vi "Version_4.9_8_on-chip_valves_for25ulSyringe_withModfied_Plunging.vi"() -> ()   [LabVIEW 2020] (continued)
                    n8528 = Wait (ms)(milliseconds to wait=w300) -> ()  [unwired: 1 out]
                  }
                  frame #3 {
                    n8529 = local write "Suction On/Off"(TRUE ("Suction On/Off")) -> ()
                  }
                  frame #4 {
                    n8530 = local read "Delay before\n1st movement\nof grid"() -> (w304:dbl)
                    n8531 = Wait (ms)(milliseconds to wait=w304) -> ()  [unwired: 1 out]
                  }
                  frame #5 {
                    n8532 = local read "No of cycles\nof up-down\nmovement"() -> (w305:dbl)
                    n8533 = for {
                      N: w305 -> [_]
                      shift-right: [w319] -> w311
                      shift-left: w313 -> [w321]
                      shift-right: [w318] -> w310
                      shift-left: w312 -> [w320]
                      shift-right: [w315] -> w307
                      shift-left: w309 -> [w317]
                      shift-right: [w314] -> w306
                      shift-left: w308 -> [w316]
                      n8534 = stacked-sequence {
                        seq-local: [w323 _ _ _ _ _] -> [_ _ _ w345 _ _]
                        seq-local: [w322 _ _ _ _ _] -> [_ _ _ w344 _ _]
                        seq-local: [_ _ w329 _ _ _] -> [_ _ _ _ _ w353]
                        seq-local: [_ _ w328 _ _ _] -> [_ _ _ _ _ w352]
                        tunnel: [_ _ _ w346 _ _] -> w319
                        tunnel: [_ _ _ w348 _ _] -> w318
                        tunnel: w321 -> [w326 _ _ _ _ _]
                        tunnel: w320 -> [w325 _ _ _ _ _]
                        tunnel: w317 -> [_ _ w331 _ _ _]
                        tunnel: w316 -> [_ _ w330 _ _ _]
                        tunnel: [_ _ _ _ _ w351] -> w315
                        tunnel: [_ _ _ _ _ w350] -> w314
                        frame #0 {
                          n8535 = VISA Write(VISA resource name=w326, write buffer="d", error in (no error)=w325) -> (VISA resource name out=w323:refnum<visa-resource-name>, error out=w322:errorcluster)  [unwired: 1 out]
                        }
                        frame #1 {
                          n8536 = local read "Duration for \nup/down\nMovement of Grid"() -> (w327:u32)
                          n8537 = Wait (ms)(milliseconds to wait=w327) -> ()  [unwired: 1 out]
                        }
                        frame #2 {
                          n8538 = stacked-sequence {
                            tunnel: w331 -> [_ w339 _]
                            tunnel: w330 -> [_ w338 _]
                            tunnel: [_ w337 _] -> w329
                            tunnel: [_ w336 _] -> w328
                            frame #0 {
                              n8539 = local read "Translation Step SIze\nwhile plunging"() -> (w332:dbl)
                              n8540 = local read "k1"() -> (w334:dbl)
                              n8541 = Decrement(x=w334) -> (x-1=w333:dbl)
                              n8542 = Multiply(x=w332, y=w333) -> (x*y=w335:dbl)
                              n8543 = local write "k2"(w333) -> ()
                              n8544 = local write "Position"(w335) -> ()
                            }
                            frame #1 {
                              w342 = 1 items=["Channel1"=1, "Channel2"=2, "Channel3"=3, "Channel4"=4] ("channel")
                              n8545 = local read "Position"() -> (w341:i32)
                              n8546 = invoke class="KCubeInertialMotor" method="MoveTo"(reference=w339, error in=w338, "channel"=w342, "position"=w341, "waitTimeout"=10000) -> (reference out=w337:refnum<k24>, error out=w336:errorcluster)  [unwired: 1 in, 4 out]
                            }
                            frame #2 {
                              n8547 = local read "Wait time for\ntranslation"() -> (w343:u32)
                              n8548 = Wait (ms)(milliseconds to wait=w343) -> ()  [unwired: 1 out]
                            }
                          }
                        }
                        frame #3 {
                          n8549 = VISA Write(VISA resource name=w345, write buffer="u", error in (no error)=w344) -> (VISA resource name out=w346:refnum<visa-resource-name>, error out=w348:errorcluster)  [unwired: 1 out]
                        }
                        frame #4 {
                          n8550 = local read "Duration for \nup/down\nMovement of Grid"() -> (w349:u32)
                          n8551 = Wait (ms)(milliseconds to wait=w349) -> ()  [unwired: 1 out]
                        }
                        frame #5 {
                          n8552 = stacked-sequence {
                            tunnel: w353 -> [_ w361 _]
                            tunnel: w352 -> [_ w360 _]
                            tunnel: [_ w359 _] -> w351
                            tunnel: [_ w358 _] -> w350
                            frame #0 {
                              n8553 = local read "Translation Step SIze\nwhile plunging"() -> (w354:dbl)
                              n8554 = local read "k2"() -> (w356:dbl)
                              n8555 = Increment(x=w356) -> (x+1=w355:dbl)
                              n8556 = Multiply(x=w354, y=w355) -> (x*y=w357:dbl)
                              n8557 = local write "k1"(w355) -> ()
                              n8558 = local write "Position"(w357) -> ()
                            }
                            frame #1 {
                              w364 = 1 items=["Channel1"=1, "Channel2"=2, "Channel3"=3, "Channel4"=4] ("channel")
                              n8559 = local read "Position"() -> (w363:i32)
                              n8560 = invoke class="KCubeInertialMotor" method="MoveTo"(reference=w361, error in=w360, "channel"=w364, "position"=w363, "waitTimeout"=10000) -> (reference out=w359:refnum<k24>, error out=w358:errorcluster)  [unwired: 1 in, 4 out]
                            }
                            frame #2 {
                              n8561 = local read "Wait time for\ntranslation"() -> (w365:u32)
                              n8562 = Wait (ms)(milliseconds to wait=w365) -> ()  [unwired: 1 out]
                            }
                          }
                        }
                      }
                    }
                  }
                  frame #6 {
                    n8563 = VISA Write(VISA resource name=w370, write buffer="p", error in (no error)=w369) -> (VISA resource name out=w368:refnum<visa-resource-name>, error out=w367:errorcluster)  [unwired: 1 out]
                    n8564 = local write "Suction On/Off"(FALSE ("Suction On/Off")) -> ()
                  }
                }
              }
              frame "Spread the deposited protein on the grid in One Line and plunge" {
                n8565 = stacked-sequence {
                  seq-local: [_ _ _ w385 _] -> [_ _ _ _ w402]
                  seq-local: [_ _ _ w384 _] -> [_ _ _ _ w401]
                  tunnel: [_ _ _ _ w400] -> w377
                  tunnel: [_ _ _ _ w399] -> w376
                  tunnel: w375 -> [_ _ _ w387 _]
                  tunnel: w374 -> [_ _ _ w386 _]
                  frame #0 {
                    n8566 = local write "Re-deposit Sample\nonto Grid"(FALSE ("Re-deposit Sample\nonto Grid")) -> ()
                    n8567 = local write "Divert Sample \nonto Grid"(TRUE ("Divert Sample \nonto Grid")) -> ()
                    n8568 = local read "Grid Deposition\nDuration"() -> (w378:u32)
                    n8569 = Wait (ms)(milliseconds to wait=w378) -> ()  [unwired: 1 out]
                  }
                  frame #1 {
                    n8570 = local write "Suction On/Off"(TRUE ("Suction On/Off")) -> ()
                  }
                  frame #2 {
                    n8571 = local read "Delay before\n1st movement\nof grid"() -> (w382:dbl)
                    n8572 = Wait (ms)(milliseconds to wait=w382) -> ()  [unwired: 1 out]
                  }
                  frame #3 {
                    n8573 = local read "No of cycles\nof up-down\nmovement"() -> (w383:dbl)
                    n8574 = for {
                      N: w383 -> [_]
                      shift-right: [w389] -> w385
                      shift-left: w387 -> [w391]
                      shift-right: [w388] -> w384
                      shift-left: w386 -> [w390]
                      n8575 = stacked-sequence {
                        tunnel: w391 -> [w396 _]
                        tunnel: w390 -> [w395 _]
                        tunnel: [w393 _] -> w389
                        tunnel: [w392 _] -> w388
                        frame #0 {
                          n8576 = VISA Write(VISA resource name=w396, write buffer="y", error in (no error)=w395) -> (VISA resource name out=w393:refnum<visa-resource-name>, error out=w392:errorcluster)  [unwired: 1 out]
                        }
                        frame #1 {
                          n8577 = local read "Duration for \nup/down\nMovement of Grid"() -> (w397:u32)
                          n8578 = Wait (ms)(milliseconds to wait=w397) -> ()  [unwired: 1 out]
                        }
                      }
                    }
                  }
                  frame #4 {
                    n8579 = VISA Write(VISA resource name=w402, write buffer="p", error in (no error)=w401) -> (VISA resource name out=w400:refnum<visa-resource-name>, error out=w399:errorcluster)  [unwired: 1 out]
                    n8580 = local write "Suction On/Off"(FALSE ("Suction On/Off")) -> ()
                  }
                }
              }
            }
          }
          event "Set - Blotting Time": Value Change {
            n8581 = event-data() -> ()  [unwired: 1 in, 6 out]
            n8582 = local read "Blotting Time"() -> (w411:dbl)
            n8583 = Format Into String(format string="%0d", w411) -> (resulting string=w410:string)  [unwired: 2 in, 1 out]
            n8584 = Concatenate Strings("t" ("string"), w410, "\r\n") -> (w408:string)
            n8585 = VISA Write(VISA resource name=w407, write buffer=w408, error in (no error)=w406) -> (VISA resource name out=w405:refnum<visa-resource-name>, error out=w404:errorcluster)  [unwired: 1 out]
          }
          event "Set - Blotting Angle": Value Change {
            n8586 = event-data() -> ()  [unwired: 1 in, 6 out]
            n8587 = local read "Blotting Angle"() -> (w421:dbl)
            n8588 = Format Into String(format string="%0d", w421) -> (resulting string=w420:string)  [unwired: 2 in, 1 out]
            n8589 = Concatenate Strings("b" ("string"), w420, "\r\n") -> (w418:string)
            n8590 = VISA Write(VISA resource name=w417, write buffer=w418, error in (no error)=w416) -> (VISA resource name out=w415:refnum<visa-resource-name>, error out=w414:errorcluster)  [unwired: 1 out]
          }
          event "Automated Blotting \nand Plunging": Value Change {
            n8591 = event-data() -> ()  [unwired: 1 in, 6 out]
            n8592 = VISA Write(VISA resource name=w428, write buffer="z", error in (no error)=w427) -> (VISA resource name out=w425:refnum<visa-resource-name>, error out=w424:errorcluster)  [unwired: 1 out]
          }
          event "Move\nGrid Up": Value Change {
            n8593 = event-data() -> ()  [unwired: 1 in, 6 out]
            n8594 = VISA Write(VISA resource name=w431, write buffer="h", error in (no error)=w432) -> (VISA resource name out=w429:refnum<visa-resource-name>, error out=w430:errorcluster)  [unwired: 1 out]
          }
          event "Move Grid \nUp Faster": Value Change {
            n8595 = event-data() -> ()  [unwired: 1 in, 6 out]
            n8596 = VISA Write(VISA resource name=w436, write buffer="x", error in (no error)=w437) -> (VISA resource name out=w434:refnum<visa-resource-name>, error out=w435:errorcluster)  [unwired: 1 out]
          }
          event "Move\nGrid Down": Value Change {
            n8597 = event-data() -> ()  [unwired: 1 in, 6 out]
            n8598 = VISA Write(VISA resource name=w441, write buffer="l", error in (no error)=w442) -> (VISA resource name out=w439:refnum<visa-resource-name>, error out=w440:errorcluster)  [unwired: 1 out]
          }
          event "Move Grid \nDown Faster": Value Change {
            n8599 = event-data() -> ()  [unwired: 1 in, 6 out]
            n8600 = VISA Write(VISA resource name=w446, write buffer="y", error in (no error)=w447) -> (VISA resource name out=w444:refnum<visa-resource-name>, error out=w445:errorcluster)  [unwired: 1 out]
          }
          event "Stop for End of \nExperiment \nand Data Writing": Value Change {
            n8601 = event-data() -> ()  [unwired: 1 in, 6 out]
            n8602 = local read "Stop for End of \nExperiment \nand Data Writing"() -> (w453:bool)
          }
          event Timeout {
            n8603 = event-data() -> ()  [unwired: 1 in, 3 out]
          }
        }
        n8604 = property class="Instr"(reference=w124, error in=w123) -> (reference out=w125:refnum<visa-resource-name>, error out=w126:errorcluster, "Serial Settings:Number of Bytes at Serial Port"=w128:u32)
        n8605 = Greater Than 0?(x=w128) -> (x > 0?=w127:bool)
        n8606 = case shown="True" w127 {
          tunnel: [w136 w151] -> w120
          tunnel: [w135 w150] -> w122
          tunnel: w125 -> [w136 w148]
          tunnel: w126 -> [w135 w147]
          tunnel: [w134 w146] -> w121
          tunnel: w131 -> [w134 w145]
          frame False {
          }
          frame True {
            (unwired) u32 20 ("byte count")
            n8607 = VISA Read(VISA resource name=w148, byte count=16, error in (no error)=w147) -> (VISA resource name out=w151:refnum<visa-resource-name>, read buffer=w144:string, error out=w150:errorcluster)  [unwired: 1 out]
            n8608 = Spreadsheet String To Array(delimiter (Tab)=",", format string="%f", spreadsheet string=w144, array type (2D Dbl)=dbl[] []) -> (array=w140:dbl[])
            n8609 = Index Array(array=w140) -> (element #1=w137:dbl, element #2=→"Ethane Temperature":dbl)  [unwired: 2 in]
            "RH (%)" <- w137
            n8610 = call "Convert from Dynamic Data5"("Dynamic Data Type"=w137) -> ("Array"=w139:dbl[])  [unwired: 3 in]
            n8611 = call-poly <vilib>:"Append Waveforms.vi"("waveform B"=w139, "waveform A"=w145) -> ("waveform out"=w146:waveform(dbl))  [unwired: 8 in, 1 out]
            "Temperature of Ethane Graph" <- w146
          }
        }
      }
      n8612 = Merge Signals(w88, w87) -> (w89:dynamicdata)
      n8613 = call "Write To Measurement File"("Signals"=w89) -> ()  [unwired: 16 in, 3 out]
      n8614 = VISA Close(VISA resource name=w71, error in (no error)=w70) -> ()  [unwired: 1 out]
      n8615 = invoke class="KCubeInertialMotor" method="StopPolling"(reference=w84, error in=w83) -> (error out=w82:errorcluster)  [unwired: 1 in, 2 out]
      n8616 = invoke class="KCubeInertialMotorControl" method="CloseDevice"(reference=w86, error in=w82) -> ()  [unwired: 1 in, 3 out]
      "Discard fluid \nprior to 1st \ndeposition" <- FALSE ("Discard fluid \nprior to 1st \ndeposition")
      "SEC On" <- FALSE ("SEC On")
      "Affinity On" <- FALSE ("Affinity On")
      "Affinity Elution On" <- FALSE ("Affinity On")
      "Suction pressure \nfor grid deposition" <- sgl 0.0 ("Suction pressure \nfor grid deposition")
      "Net Elution \nVolume" <- 0.0 ("Net Elution \nVolume")
      "Pause Elution" <- FALSE ("Pause Elution")
    }
    frame #1 {
      # "Switch off the LEDs"
      n8617 = local write "Start the Process"(FALSE ("Start the Process")) -> ()
      n8618 = local write "Stop for End of \nExperiment \nand Data Writing"(FALSE ("Stop for End of \nExperiment \nand Data Writing")) -> ()
      n8619 = local write "Stopper that ends \nthe main loops"(FALSE ("Stopper that ends \nthe main loops")) -> ()
    }
  }
  "Volume being Injected \nin this process" <- 0.0 ("Volume being Injected \nin this process")
  "Total Volume \nbeing Injected" <- 0.0 ("Total Volume being Injected")
  "Volume being Injected \ntill the end of previous \nprocess" <- 0.0 ("Volume being Injected \ntill the end of previous \nprocess")
  "Pause Data Collection" <- TRUE ("Pause Data Collection")
  "Stopper that ends \nthe main loops" <- FALSE ("Stopper that ends \nthe main loops")
  "Initial Plunger Position" <- 0 ("Initial Plunger Position")
  "True Volume being \ninjected in this\nprocess" <- 0.0
  "Affinity Elution \nis Approaching" <- FALSE ("Affinity Elution \nis Approaching")
